vi "VisionTopPortOld.vi"(7 "error in":errorcluster) -> (20 "Histogram (Histogram 1)":u32[][](array[numeric]), 27 "error out":errorcluster)   [LabVIEW 2019]
uses:
  <vilib>/vision/NI_Vision_Development_Module.lvlib
panel:
  in  "x*y":dbl
  in  "y":dbl=1.4 format="%#_13g"
  in  "Minimal Score":dbl=400.0 format="%.2f"
  out "Shape Report (calibrated)":T1(array[cluster]) {"Score" format="%.2f"; "Centroid"."y" format="%.2f"; "Centroid"."x" format="%.2f"}
  out "Image Out":T2(plugin-control)
  out "Histogram Graph":u32[][](graph)
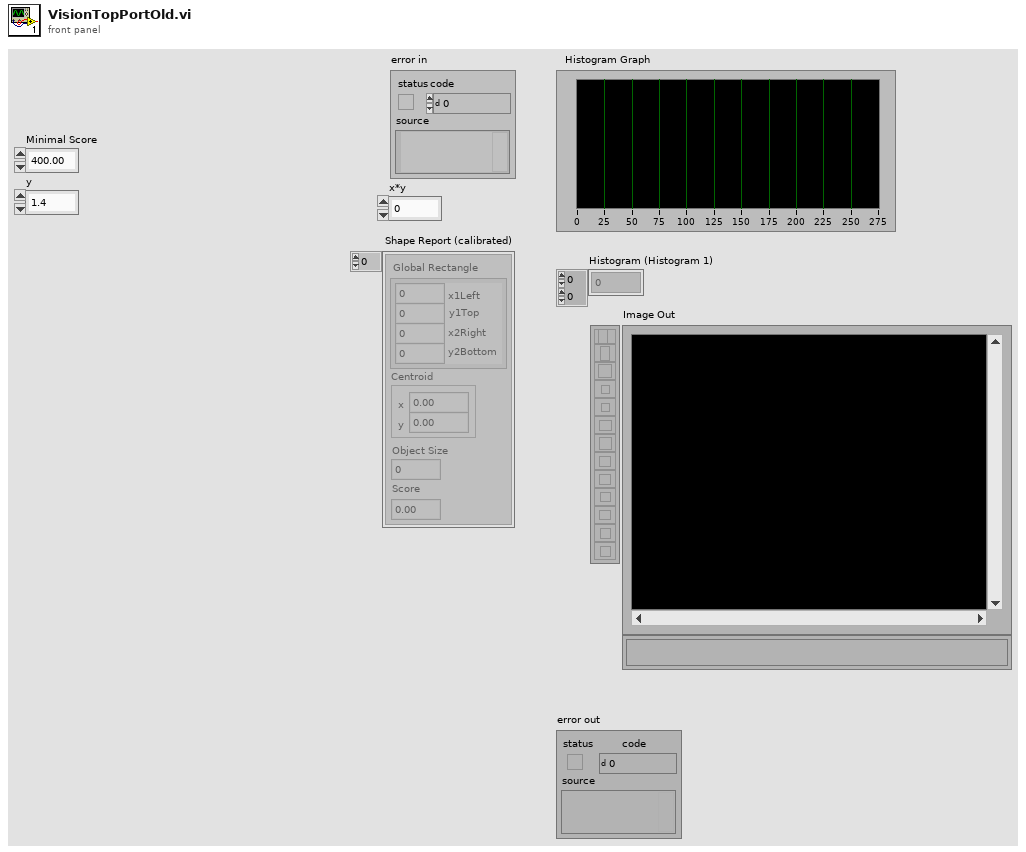
[diagram p1: front panel]
types:
  T1 = cluster{"Global Rectangle":cluster{"x1Left":i32, "y1Top":i32, "x2Right":i32, "y2Bottom":i32}, "Centroid":cluster{"x":sgl, "y":sgl}, "Object Size":u32, "Score":dbl}[]
  T2 = typedef "IMAQ Image.ctl" = refnum<image>
  T3 = cluster{"Measurement Parameter":i32, "Range Lower Value":dbl, "Range Upper Value":dbl, "Range":bool, "Measurement Type":bool}[]
  T4 = enum32{"AutoM", "Close", "Dilate", "Erode", "Gradient", "Gradient in", "Gradient out", "HitMiss", "Open", "PClose", "POpen", "Thick", "Thin"}
  T5 = cluster{"Global Rectangle":i32[], "Contours":cluster{"ID":enum32{"External", "Internal"}, "Type":u32, "Coordinates":i32[]}[]}
  T6 = cluster{"Minimal Value":sgl, "Maximal Value":sgl, "Mean Value":sgl, "Standard  Variation":sgl, "Area (pixels)":i32}
  T7 = cluster{"histogram":u32[], "Minimal Value":sgl, "Maximal Value":sgl, "Starting Value":sgl, "Interval Width":sgl, "Mean Value":sgl, "Standard  Variation":sgl, "Area (pixels)":i32}
  T8 = typedef "Image Type" = u32
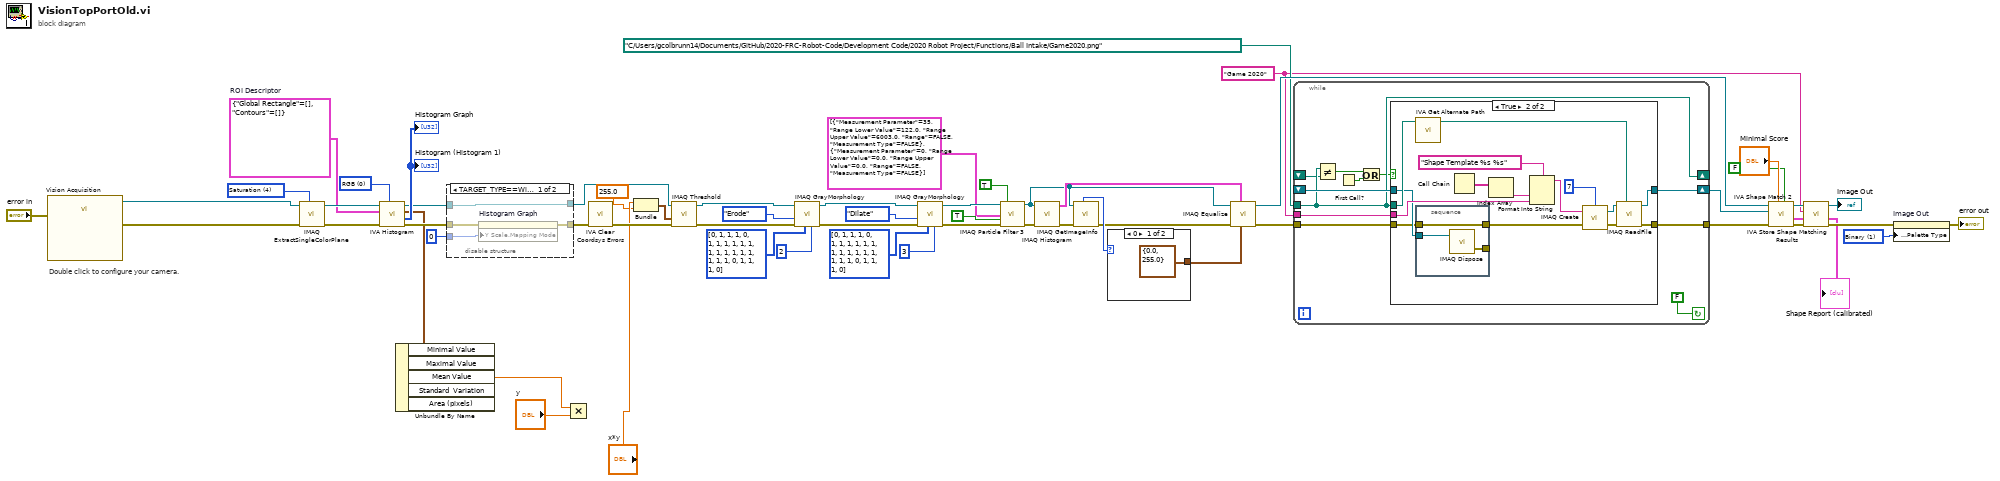
[diagram p0: block diagram]
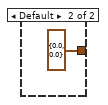
[diagram p3: hidden frame]
diagram:
  w8 = u32 1 items=["Grayscale", "Binary", "Gradient", "Rainbow", "Temperature", "User Defined", "Binary 16 Bit", "Gradient 16 Bit", "Rainbow 16 Bit", "Temperature 16 Bit", "User Defined 16 Bit"] ("Palette Type")
  w12 = "Game 2020" ("Step Name")
  w53 = u16 0 items=["RGB", "HSL", "HSV", "HSI"] ("Color Mode")
  w51 = T5 {"Global Rectangle"=[], "Contours"=[]}  # ROI Descriptor
  w58 = 4 items=["Red", "Green", "Blue", "Hue", "Saturation", "Luminance", "Value", "Intensity"] ("Color Plane")
  # "Double click to configure your camera."
  n1 = call "Vision Acquisition"("error in"="error in") -> ("Image Out"=w57:T2, "error out"=w56:errorcluster)  [unwired: 25 in]
  n2 = call "IMAQ ExtractSingleColorPlane"("Color Plane"=w58, "error in (no error)"=w56, "Image Src"=w57) -> ("error out"=w50:errorcluster, "Image Dst Out"=w55:T2)  [unwired: 1 in, 6 out]
  n3 = call <vilib>:"IVA Histogram.vi"("Color Mode"=w53, "error in (no error)"=w50, "ROI Descriptor"=w51, "Image In"=w55) -> ("error out"=w54:errorcluster, "Histograms"=→"Histogram Graph" →"Histogram (Histogram 1)":u32[][], "Statistics"=w7:T6, "Image Out"=w49:T2)  [unwired: 4 out]
  n4 = Unbundle By Name(w7) -> ("Mean Value"=w5:sgl)  [unwired: 4 out]
  n5 = disable-structure "Conditional Disable Structure" shown="TARGET_TYPE==Windows" {
    disable-tunnel: w54 -> [w63 w64]
    disable-tunnel: [w62 w64] -> w47
    disable-tunnel: w49 -> [w61 w65]
    disable-tunnel: [w61 w65] -> w46
    disable-tunnel: u8 0 ("Y Scale.Mapping Mode") -> [w60 _]
    frame condition #0 {
      n6 = property on="Histogram Graph" class="WFGraph (strict)"(error in=w63, "Y Scale.Mapping Mode"=w60) -> (error out=w62:errorcluster)  [unwired: 1 in, 1 out]
    }
    frame condition #1 (active) {
    }
  }
  n7 = Multiply(x=w5, y="y") -> ()  [unwired: 1 out]
  n8 = call <vilib>:"IVA Clear Coordsys Errors.vi"("error in (no error)"=w47) -> ("error out"=w45:errorcluster)  [unwired: 10 in]
  n9 = Bundle("x*y"="x*y", "Upper value"=sgl 255.0) -> (w4:cluster{"x*y":dbl, "Upper value":sgl})  [unwired: 1 in]
  n10 = call "IMAQ Threshold"("error in (no error)"=w45, "Range"=w4, "Image Src"=w46) -> ("error out"=w41:errorcluster, "Image Dst Out"=w42:T2)  [unwired: 3 in, 4 out]
  n11 = call "IMAQ GrayMorphology"("Number of iterations (1)"=2, "Structuring Element"=i32[][] [[0, 1, 1, 1, 0], [1, 1, 1, 1, 1], [1, 1, 1, 1, 1], [1, 1, 1, 1, 1], [0, 1, 1, 1, 0]], "error in (no error)"=w41, "Operation"=T4."Erode", "Image Src"=w42) -> ("error out"=w36:errorcluster, "Image Dst Out"=w37:T2)  [unwired: 2 in, 3 out]
  n12 = call "IMAQ GrayMorphology"("Number of iterations (1)"=3, "Structuring Element"=i32[][] [[0, 1, 1, 1, 0], [1, 1, 1, 1, 1], [1, 1, 1, 1, 1], [1, 1, 1, 1, 1], [0, 1, 1, 1, 0]], "error in (no error)"=w36, "Operation"=T4."Dilate", "Image Src"=w37) -> ("error out"=w31:errorcluster, "Image Dst Out"=w32:T2)  [unwired: 2 in, 3 out]
  n13 = call "IMAQ Particle Filter 3"("Image Src"=w32, "Connectivity 4/8 (8)"=TRUE, "Selection Values"=T3 [{"Measurement Parameter"=35, "Range Lower Value"=122.0, "Range Upper Value"=6003.0, "Range"=FALSE, "Measurement Type"=FALSE}, {"Measurement Parameter"=0, "Range Lower Value"=0.0, "Range Upper Value"=0.0, "Range"=FALSE, "Measurement Type"=FALSE}], "Keep/Remove Particles (F)"=TRUE ("Keep/Remove Particles"), "error in (no error)"=w31) -> ("Image Dst Out"=w26:T2, "error out"=w28:errorcluster)  [unwired: 4 in, 5 out]
  n14 = call "IMAQ Histogram"("error in (no error)"=w28, "Image"=w26) -> ("error out"=w25:errorcluster, "Histogram Report"=w29:T7)  [unwired: 3 in, 5 out]
  n15 = call "IMAQ GetImageInfo"("error in (no error)"=w25, "Image"=w26) -> ("error out"=w24:errorcluster, "Image Type"=w27:T8)  [unwired: 8 out]
  n16 = case shown="0" w27 {
    tunnel: [cluster{"Minimum":sgl, "Maximum":sgl} {"Minimum"=0.0, "Maximum"=255.0} ("Range") cluster{"Minimum":sgl, "Maximum":sgl} {"Minimum"=0.0, "Maximum"=0.0} ("Range")] -> w23
    frame 0 {
    }
    frame Default {
    }
  }
  n17 = call "IMAQ Equalize"("Range"=w23, "Histogram Report"=w29, "error in (no error)"=w24, "Image Src"=w26) -> ("error out"=w15:errorcluster, "Image Dst Out"=w20:T2)  [unwired: 2 in, 4 out]
  n18 = while {
    shift-right: [w78] -> w13
    shift-left: _ -> [w77]
    tunnel: [w75] -> w14
    tunnel: w15 -> [w74]
    tunnel: path "C:/Users/gcolbrunn14/Documents/GitHub/2020-FRC-Robot-Code/Development Code/2020 Robot Project/Functions/Ball Intake/Game2020.png" ("Template Path") -> [w72]
    tunnel: w12 -> [w73]
    shift-right: [w72] -> _
    shift-left: _ -> [w71]
    stop <- FALSE continue-if-true
    n19 = Not Equal?(x=w72, y=w71) -> (x != y?=w69:bool)
    n20 = First Call?() -> (First Call?: T/F=w70:bool)
    n21 = Or(x=w69, y=w70) -> (x .or. y?=w68:bool)
    n22 = case shown="True" w68 {
      tunnel: [w80 w92] -> w78
      tunnel: w77 -> [w80 w83]
      tunnel: [w79 w90] -> w75
      tunnel: w74 -> [w79 w82]
      tunnel: w72 -> [_ w85]
      tunnel: w73 -> [_ w86]
      frame False {
      }
      frame True {
        n23 = call <vilib>:"IVA Get Alternate Path.vi"("Path In"=w85) -> ("Path Out"=w84:path)  [unwired: 10 out]
        n24 = stacked-sequence {
          tunnel: w83 -> [w98]
          tunnel: w82 -> [w97]
          tunnel: [w97] -> w81
          tunnel: [w96] -> _
          frame #0 {
            n25 = call "IMAQ Dispose"("Image"=w98) -> ("error out"=w96:errorcluster)  [unwired: 2 in, 3 out]
          }
        }
        n26 = Call Chain() -> (call chain=w88:string[])
        n27 = Index Array(array=w88) -> (element=w87:string)  [unwired: 1 in]
        n28 = Format Into String(format string="Shape Template %s %s" ("Image Name"), w87, w86) -> (resulting string=w95:string)  [unwired: 2 in, 1 out]
        n29 = call "IMAQ Create"("Border Size"=7, "Image Name"=w95, "error in (no error)"=w81) -> ("New Image"=w93:T2, "error out"=w91:errorcluster)  [unwired: 1 in, 1 out]
        n30 = call "IMAQ ReadFile"("File Path"=w84, "error in (no error)"=w91, "Image"=w93) -> ("error out"=w90:errorcluster, "Image Out"=w92:T2)  [unwired: 2 in, 5 out]
      }
    }
  }
  n31 = call <vilib>:"IVA Shape Match 2.vi"("Scale Invariance"=FALSE, "Minimal Score"="Minimal Score", "error in (no error)"=w14, "Template"=w13, "Image Src"=w20) -> ("error out"=w19:errorcluster, "Shape Report"=w18:T1, "Image Out"=w17:T2)  [unwired: 4 out]
  n32 = call <vilib>:"IVA Store Shape Matching Results.vi"("error in (no error)"=w19, "Shape Report"=w18, "Step Name"=w12, "Image in"=w17) -> ("error out"=w11:errorcluster, "Shape Report (calibrated)"=→"Shape Report (calibrated)":T1, "Image dup"=→"Image Out":T2)  [unwired: 5 out]
  n33 = property on="Image Out" class="ImageControl"(error in=w11, "Palette:Palette Type"=w8) -> (error out=→"error out":errorcluster)  [unwired: 1 in, 1 out]
